vi "Read ADC.vi"(8 "error in (no error)":errorcluster, 10 "Canal":string, 11 "UI Actor in":refnum<class "UI Actor.lvclass">) -> (0 "error out":errorcluster, 3 "UI Actor out":refnum<class "UI Actor.lvclass">)   [LabVIEW 2020, in "UI Actor.lvlib" / "UI Actor.lvclass"]
uses:
  UI Actor.lvclass
  UI Actor.lvclass/UI Actor.ctl
  Abstract/Serial Device/Serial Device.lvclass
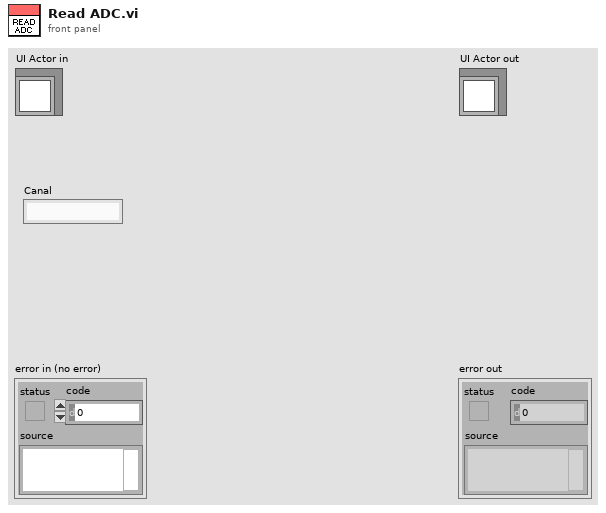
[diagram p1: front panel]
types:
  T1 = typedef "Control 1.ctl" = string
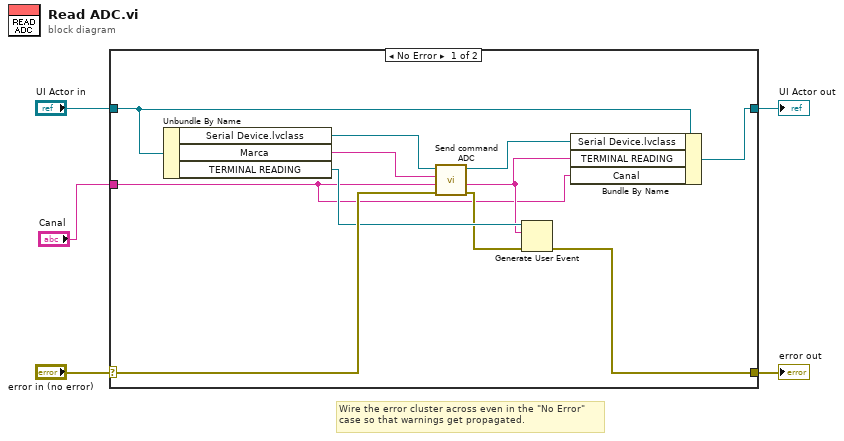
[diagram p0: block diagram]
diagram:
  # "Wire the error cluster across even in the \"No Error\"\ncase so that warnings get propagated."
  n1 = case shown="No Error" "error in (no error)" {
    selector: "error in (no error)" -> [w12 w18]
    tunnel: [w7 w18] -> w4
    tunnel: [w14 w17] -> w2
    tunnel: "UI Actor in" -> [w15 w17]
    tunnel: "Canal" -> [w6 _]
    frame No Error {
      n2 = Unbundle By Name(w15) -> ("Serial Device.lvclass"=w16:refnum<class "Serial Device.lvclass">, "Marca"=w11:T1, "TERMINAL READING"=w10:refnum<user-event>)
      n3 = call-dynamic "Send command ADC.vi"("error in (no error)"=w12, "Canal"=w6, "Marca"=w11, "object in"=w16) -> ("error out"=w8:errorcluster, "Expected response"=w9:string, "object out"=w13:refnum<class "Serial Device.lvclass">)  [unwired: 4 in, 1 out]
      n4 = Generate User Event(user event=w10, event data cluster=w9, error in=w8) -> (error out=w7:errorcluster)  [unwired: 1 in, 1 out]
      n5 = Bundle By Name(cluster=w15, "Serial Device.lvclass"=w13, "TERMINAL READING"=w9, "Canal"=w6) -> (w14:refnum<class "UI Actor.lvclass">)
    }
    frame Error {
    }
  }
  "error out" <- w4
  "UI Actor out" <- w2
